vi "IIR Filter with I.C. (DBL).vi"(5 "Initial Y Conditions":dbl[](array[numeric]), 6 "Initial X Conditions":dbl[](array[numeric]), 7 "Forward Coefficients":dbl[](array[numeric]), 9 "Reverse Coefficients":dbl[](array[numeric]), 10 "X":dbl[](array[numeric])) -> (0 "Final X Conditions":dbl[](array[numeric]), 1 "Final Y Conditions":dbl[](array[numeric]), 2 "error":i32, 3 "Filtered X":dbl[](array[numeric]))   [LabVIEW 2010, in "NI_AALBase.lvlib"]
doc: "Filters the input sequence <B>X</B> using the direct form IIR filter specified by <B>Reverse Coefficients</B> and <B>Forward Coefficients</B>. You can use this VI to process blocks of continuous data. This VI is similar to the IIR Filter VI except that you specify the initial conditions for this VI. Wire data to the <B>X</B> input to determine the polymorphic instance to use or manually select the instance."
uses:
  NI_AALBase.lvlib
  lvanlys.dll
panel:
  # "IIR Filter with I.C."
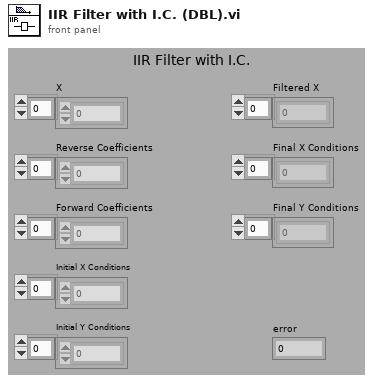
[diagram p1: front panel]
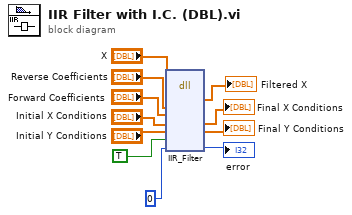
[diagram p0: block diagram]
diagram:
  n1 = dll-call lib="C:/Program Files/National Instruments/LabVIEW 2010/resource/lvanlys.*" fn="IIR_Filter"("X"="X", "Reverse Coefficients"="Reverse Coefficients", "Forward Coefficients"="Forward Coefficients", "Initial X Conditions"="Initial X Conditions", "Initial Y Conditions"="Initial Y Conditions", TRUE, 0) -> ("X"=→"Filtered X":dbl[], "Initial X Conditions"=→"Final X Conditions":dbl[], "Initial Y Conditions"=→"Final Y Conditions":dbl[], →"error":i32)  [unwired: 7 in, 2 out]
